vi "getAllChannels.vi"(8 "error in (no error)":errorcluster, 11 "Instrument.Amplifier in":refnum<class "Instrument.Amplifier.lvclass">) -> (0 "error out":errorcluster, 2 "allChannelProperties":variant, 3 "Instrument.Amplifier out":refnum<class "Instrument.Amplifier.lvclass">)   [LabVIEW 2019, in "Instrument.Amplifier.lvclass"]
uses:
  Instrument.Amplifier.lvclass
  Amplifier.Commands--Enum.ctl
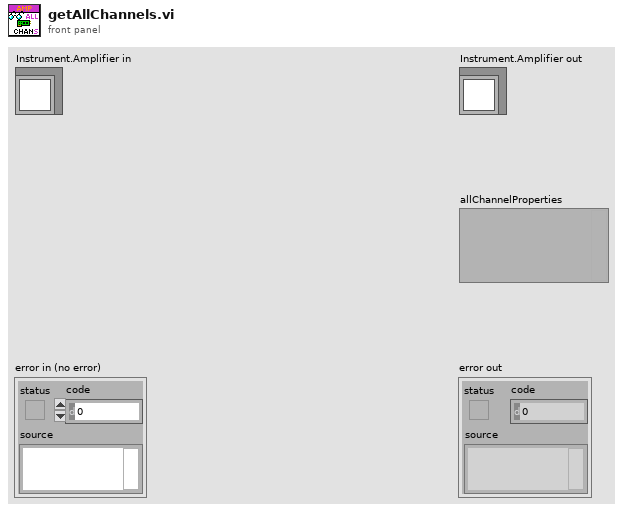
[diagram p1: front panel]
types:
  T1 = typedef "Instrument.Amplifier.lvclass/Amplifier.Commands--Enum.ctl" = enum16{"getChannel", "getAllChannels", "setChannel", "setAllChannels"}
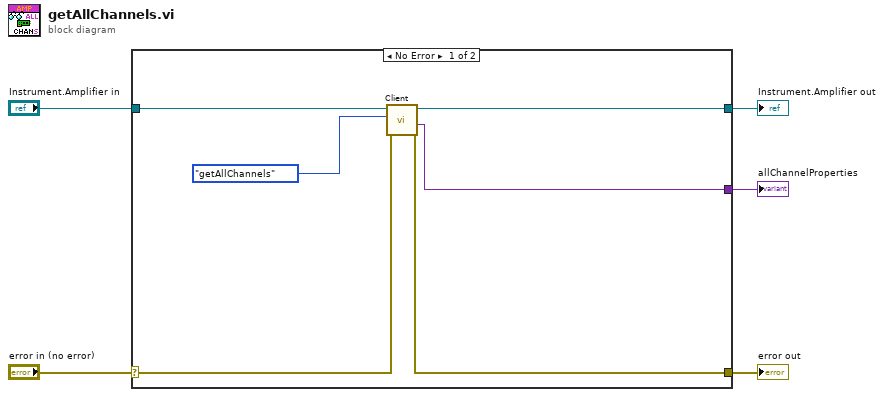
[diagram p0: block diagram]
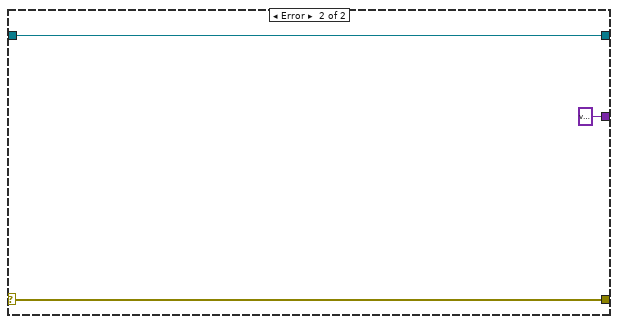
[diagram p2: hidden frame]
diagram:
  n1 = case shown="No Error" "error in (no error)" {
    selector: "error in (no error)" -> [w10 w14]
    tunnel: [w8 w14] -> w4
    tunnel: [w11 w13] -> w2
    tunnel: "Instrument.Amplifier in" -> [w6 w13]
    tunnel: [w9 variant ("Data out")] -> w1
    frame No Error {
      n2 = call-dynamic "Client.vi"("error in (no error)"=w10, "Command in"=Amplifier.Commands--Enum."getAllChannels" ("Commands"), "Instrument in"=w6) -> ("error out"=w8:errorcluster, "Data out"=w9:variant, "Instrument out"=w11:refnum<class "Instrument.Amplifier.lvclass">)  [unwired: 5 in, 1 out]
    }
    frame Error {
    }
  }
  "error out" <- w4
  "Instrument.Amplifier out" <- w2
  "allChannelProperties" <- w1
